vi "Edit Connector Pane - Multiple Converter.vi"(11 "error in":errorcluster) -> (15 "error out":errorcluster)   [LabVIEW 2021, in "Converter.lvlib"]
uses:
  Converter.lvlib
  Converter Reusables/Converter Reusables.lvlib
  Path Functions/Path Functions.lvlib
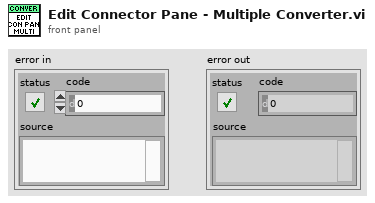
[diagram p1: front panel]
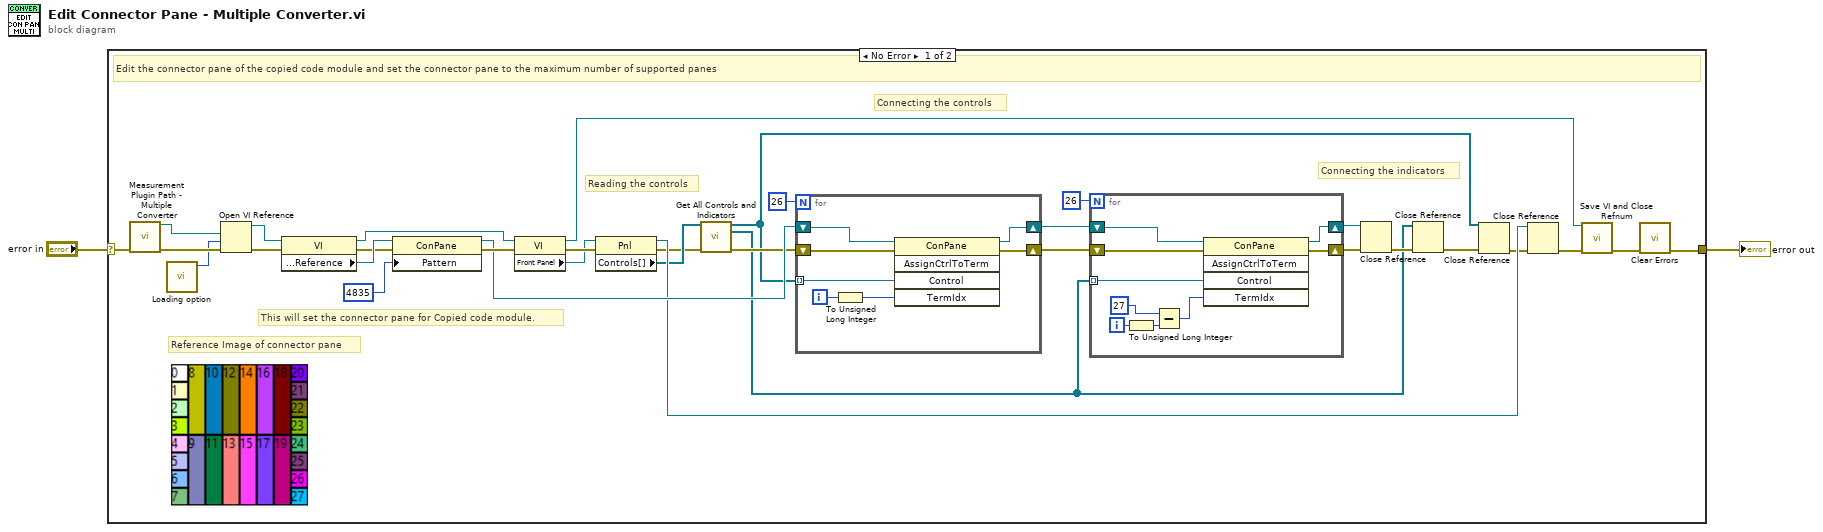
[diagram p0: block diagram]
diagram:
  n1 = case shown="No Error" "error in" {
    selector: "error in" -> [w6 w52]
    tunnel: [w7 w52] -> w1
    frame No Error {
      # "Reference Image of connector pane"
      # "Connecting the indicators"
      # "Connecting the controls"
      # "Reading the controls"
      # "This will set the connector pane for Copied code module."
      # "Edit the connector pane of the copied code module and set the connector pane to the maximum number of supported panes"
      n2 = call "Measurement Plugin Path - Multiple Converter.vi"("error in"=w6) -> ("new code module"=w4:path, "error out"=w5:errorcluster)  [unwired: 2 in, 11 out]
      n3 = call "Loading option.vi"() -> ("options"=w3:i32)  [unwired: 11 in]
      n4 = Open VI Reference(vi path=w4, options=w3, error in (no error)=w5) -> (vi reference=w24:refnum<vi>, error out=w30:errorcluster)  [unwired: 1 in, 2 out]
      n5 = property class="VI"(reference=w24, error in=w30) -> (reference out=w35:refnum<vi>, error out=w31:errorcluster, "Connector Pane:Reference"=w33:refnum<vi>)
      n6 = property class="ConPane"(reference=w33, error in=w31, "Pattern"=u32 4835) -> (reference out=w29:refnum<vi>, error out=w32:errorcluster)
      n7 = property class="VI"(reference=w35, error in=w32) -> (reference out=w20:refnum<vi>, error out=w34:errorcluster, "Front Panel"=w21:refnum<vi>)
      n8 = property class="Pnl"(reference=w21, error in=w34) -> (reference out=w19:refnum<vi>, error out=w8:errorcluster, "Controls[]"=w9:refnum<vi>[])
      n9 = call "Get All Controls and Indicators.vi"("controls[]"=w9, "error in"=w8) -> ("controls[]"=w14:refnum<vi>[], "indicators[]"=w10:refnum<vi>[], "error out"=w17:errorcluster)  [unwired: 11 in]
      n10 = for {
        N: 26 -> [_]
        tunnel: w14 -> [w39] mode=indexing
        shift-right: [w38] -> w26
        shift-left: w17 -> [w41]
        shift-right: [w40] -> w28
        shift-left: w29 -> [w42]
        i -> [w37]
        n11 = To Unsigned Long Integer(number=w37) -> (unsigned 32bit integer=w36:u32)
        n12 = invoke class="ConPane" method="AssignCtrlToTerm"(reference=w42, error in=w41, "Control"=w39, "TermIdx"=w36) -> (reference out=w40:refnum<vi>, error out=w38:errorcluster)  [unwired: 1 in, 3 out]
      }
      n13 = for {
        N: 26 -> [_]
        tunnel: w10 -> [w48] mode=indexing
        shift-right: [w47] -> w25
        shift-left: w26 -> [w50]
        shift-right: [w49] -> w27
        shift-left: w28 -> [w51]
        i -> [w46]
        n14 = To Unsigned Long Integer(number=w46) -> (unsigned 32bit integer=w43:u32)
        n15 = Subtract(x=u32 27 ("Terminal Index"), y=w43) -> (x-y=w44:u32)
        n16 = invoke class="ConPane" method="AssignCtrlToTerm"(reference=w51, error in=w50, "Control"=w48, "TermIdx"=w44) -> (reference out=w49:refnum<vi>, error out=w47:errorcluster)  [unwired: 1 in, 3 out]
      }
      n17 = Close Reference(reference=w27, error in (no error)=w25) -> (error out=w11:errorcluster)
      n18 = Close Reference(reference=w10, error in (no error)=w11) -> (error out=w12:errorcluster)
      n19 = Close Reference(reference=w14, error in (no error)=w12) -> (error out=w13:errorcluster)
      n20 = Close Reference(reference=w19, error in (no error)=w13) -> (error out=w18:errorcluster)
      n21 = call "Save VI and Close Refnum.vi"("vi refnum"=w20, "error in"=w18) -> ("error out"=w22:errorcluster)  [unwired: 13 in]
      n22 = call <vilib>:"Clear Errors.vi"("error in (no error)"=w22) -> ("error out"=w7:errorcluster)  [unwired: 5 in, 1 out]
    }
    frame Error {
    }
  }
  "error out" <- w1
